vi "0x51_Cmd_read_description_one_table_parameter_(SubVI).vi"(10 "NumberTableParam":i32 format="%0d", 11 "String in":string) -> (3 "String out":string)   [LabVIEW 2017, in "LV_Unicorn.lvlib"]
uses:
  LV_Unicorn.lvlib
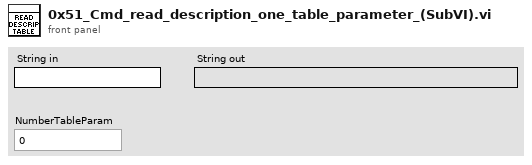
[diagram p1: front panel]
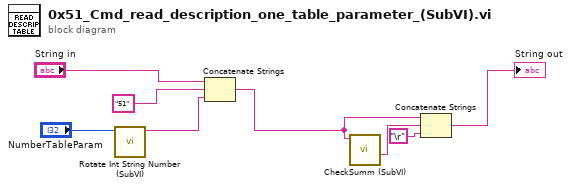
[diagram p0: block diagram]
diagram:
  n1 = call "Rotate Int String Number (SubVI).vi"("Int Number In"="NumberTableParam") -> ("Orig String"=w2:string)  [unwired: 8 in, 2 out]
  n2 = Concatenate Strings("String in", "51" ("string"), w2) -> (w3:string)
  n3 = call "CheckSumm (SubVI).vi"("Input String"=w3) -> ("CheckSumm"=w4:string)  [unwired: 7 in, 3 out]
  n4 = Concatenate Strings(w3, w4, "\r") -> (→"String out":string)
